vi "SprachEditor.vi"() -> ()   [LabVIEW 2020, in "Sprachverwaltung.lvlib"]
uses:
  Sprachverwaltung.lvlib
  Allgemein/Sprachauswahl native.ctl
  Visualisierungs Elemente/Button.ctl
  Seiten.ctl
  FGV Aktion Tabelle zerlegen.ctl
  Seiten/System Einstellungen V2/Aktioen FGV System Konstanten.ctl
  Allgemein/allgemeine Sub-VIs.lvlib
  Seiten/System Einstellungen V2/System Einstellungen V2.lvlib
panel:
  in  "Registerkarte":enum32{"Deutsch", "English"}(tab)
  out "Deutsch":string[](array[string])
  out "English":string[](array[string]) caption="Englisch"
  in  "Bearbeitungsspalte":string[](array[string])
  in  "Seiten":T1 caption="Seiten:"
  in  "Save":T2 caption="Abbrechen"
  in  "Cancel":T2 caption="Abbrechen"
  in  "Sprache":T3 caption="Bitte wählen Sie eine Sprache:" items=["Français"=2, "Italiano"=3, "Castellano"=4, "Polski"=5]
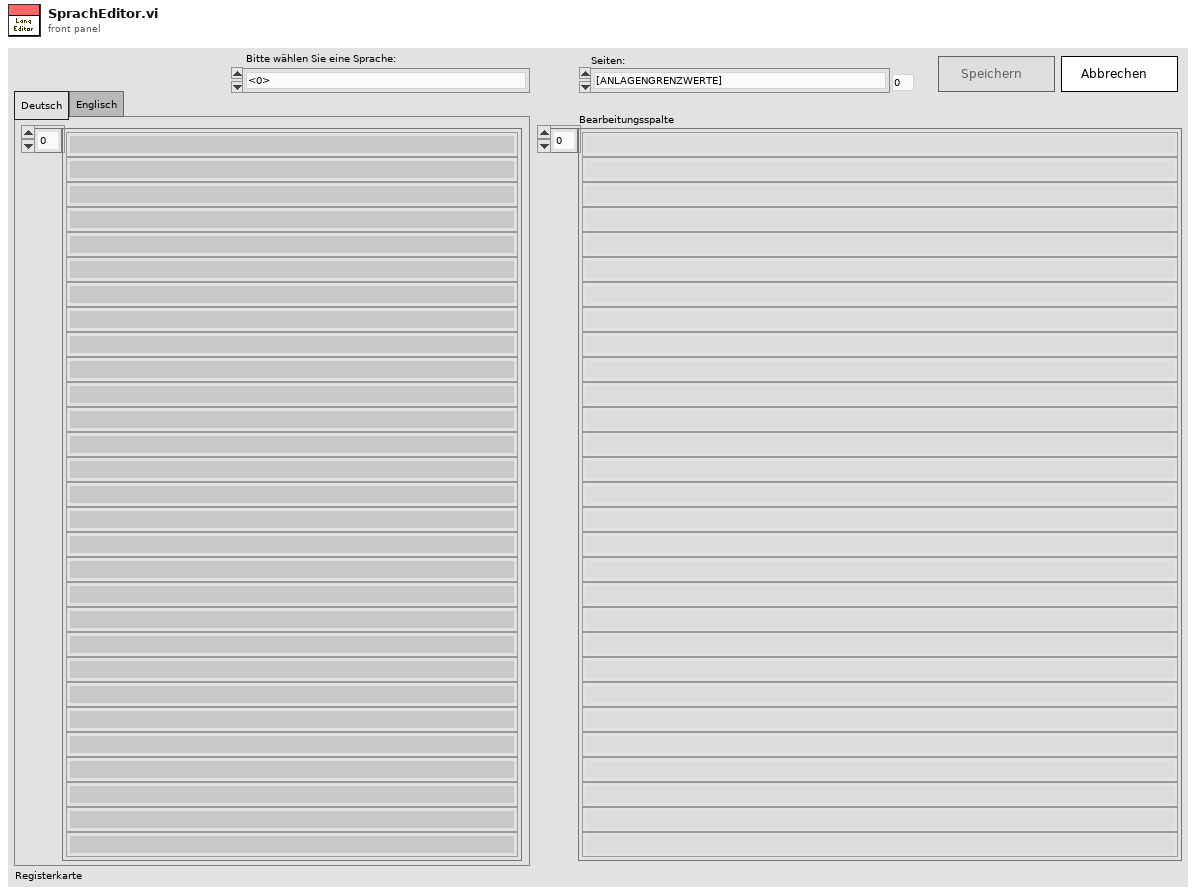
[diagram p1: front panel]
types:
  T1 = typedef "Sprachverwaltung.lvlib/Seiten.ctl" = enum16{"[ANLAGENGRENZWERTE]", "[LOG KONFIG]", "[GASZUORDNUNG]", "[ANLAGENÜBERSICHT]", "[GRAFIK]", "[CONFIG DIAGRAMME]", "[KONFIGURATION FTIR]", "[GASLISTE VERGLEICHEN]", "[ALGEBRAIC KONFIG]", "[FTIR DIAGNOSE]", "[ERWEITERTE KONFIG]", "[KONFIG AK]", "[STATUS STEUERUNG]", "[PID PARAMETER DRUCK-REGLER]", "[DICHTHEITSTEST]", "[T90 KONFIG]", "[T90]", "[HINTERGRUND]", "[SYSTEM EINSTELLUNGEN V2]", "[COPYRIGHT]", "[STATUSÜBERSICHT]", "[PASSWORTVERWALTUNG]", "[PASSWORT AENDERN]", "[FUNKTIONSTASTEN]", "[PNS]", "[DIAG PNS]", "[RUNTIME MENUE]", "[FAS06]", "[PERMANENT BEREICH]", "[RUNTIME BEENDEN]", "[SPEICHERN]", "[STOERMELDUNGEN]", "[STOERMELDEPUFFER]", "[STOERMELDE-KONFIG]", "[STOERMELDUNGSDATEI]", "[ERWEITERTE GASLISTE]", "[LINEARISIERUNG FTIR]", "[ARN TEST]", "[ARN PROTOKOLL]", "[FEHLER STEUERUNG]", "[POLYNOMKOEFFIZIENTEN]", "[KONFIG LINEARITY VERIFICATION]", "[AUTO LIN VERIFICATION]", "[GRAPHIK KURVEN]", "[EPA DICHTHEITSTEST]", "[REZEPT LADEN]", "[REZEPTWECHSEL]", "[DIAG ZYKLUSZEIT]", "[EPA KONTROLLE PARAMETER]", "[KONFIG GASTEILER]", "[KALIBRIERDATEN LADEN]", "[KONTROLLE PARAMETER VOR LIN]", "[KONFIGURATION KALIBRIERGASE]", "[INTERFERENCE VERIFICATION]", "[INTERFERENCE VERIFICATION 375]", "[INTERFERENCE PROTOKOLL 375]", "[INTERFERENCE PROTOKOLL]", "[INTERFERENCE HILFE]", "[SPUELEN]", "[GASTEILER SPUELEN]", "[GASTEILER KALIBRIEREN]", "[SENSOR KONFIGURATION]", "[KONFIGURATION PMA]", "[KALIBRIERDATEN]", "[KONFIGURATION FID]", "[ABB MANUELL KALIBRIEREN]", "[PMA MANUELL KALIBRIEREN]", "[SPRACHAUSWAHL]", "[SYS LOG HISTORY]", "[SYS LOG STATUS]", "[PNS UEBERSICHT]\t", "[CG TEST]", "[KONFIG CG CHECK]", "[HOVA MAIN]", "[HORIBA GDC]", "[BACKUP]", "[SPAN FAKTOREN]", "[CG POPUP]", "[AUTO CALIBRATION]", "[LIN V2]", "[O2 LEAKTEST]", "[CG TEST RESULT]", "[GASTEILER ABWEICHUNG]", "[EPA LIN CHECK PROTOKOLL]", "[LIN CHECK PROTOKOLL]", "[LEAK CHECK PROTOKOLL]", "[O2 LEAK PROTOKOLL]", "[HANG UP PROTOKOLL]", "[T90 PROTOKOLL]", "[SPRACHEDITOR]", "[SYSLOG CRIO MESSAGES]", "[SYSLOG PC MESSAGES]", "[SYSLOG PROPERTIES MESSAGES]", "[T90 EPA]", "[T90 EPA PDF]", "[SCHEDULER]", "[HINTERGRUND V2]", "[CG TEST PDF]", "[CHILLER EPA TEST]", "[CHILLER EPA PROTOKOLL]", "[FID O2 EPA TEST]", "[FID O2 EPA PROTOKOLL]", "[DRIFT EPA TEST]", "[DRIFT EPA PROTOKOLL]", "[PRE EPA TEST]", "[PRE EPA PROTOKOLL]", "[FID OPTIMIZATION]", "[FID OPTIMIZATION PDF]", "[FID RESPONSE FAKTOR]"}
  T2 = typedef "Button.ctl" = bool
  T3 = typedef "Sprachverwaltung.lvlib/Sprachauswahl native.ctl" = u16
  T4 = typedef "Sprachverwaltung.lvlib/FGV Aktion Tabelle zerlegen.ctl" = enum16{"laden", "vereinzeln", "speichern"}
  T5 = enum8{"Enabled", "Disabled", "Disabled and Grayed Out"}
  T6 = typedef "LVStringsAndValuesArrayTypeDef_U16.ctl" = cluster{"String":string, "Value":u16}[]
  T7 = typedef "System Einstellungen V2.lvlib/Aktioen FGV System Konstanten.ctl" = enum16{"lesen", "laden", "speichern", "Sprache"}
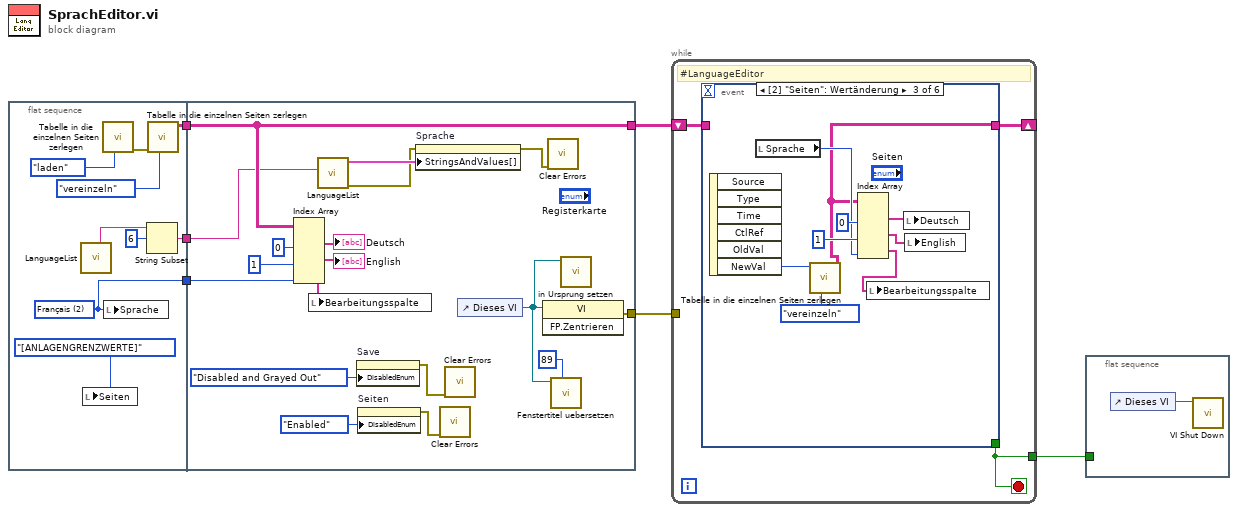
[diagram p0: block diagram]
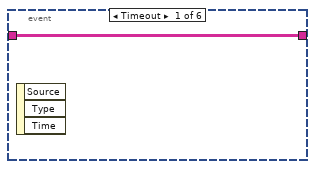
[diagram p2: hidden frame]
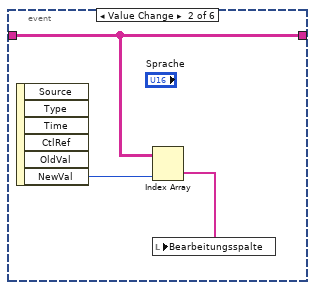
[diagram p3: hidden frame]
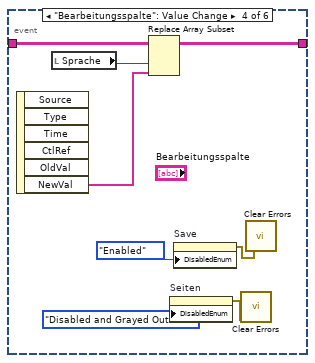
[diagram p4: hidden frame]
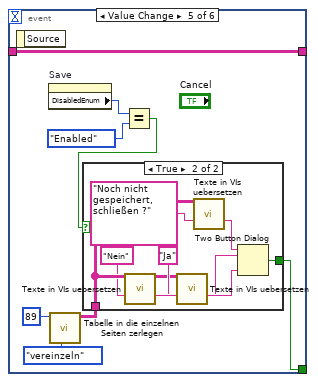
[diagram p5: hidden frame]
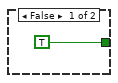
[diagram p6: hidden frame]
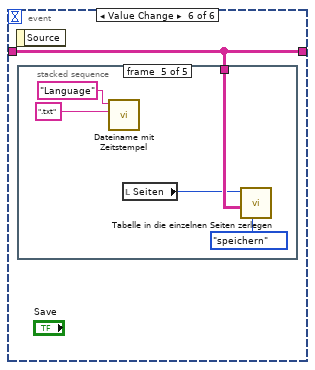
[diagram p7: hidden frame]
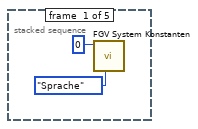
[diagram p8: hidden frame]
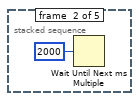
[diagram p9: hidden frame]
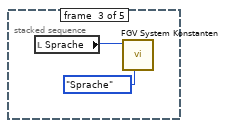
[diagram p10: hidden frame]
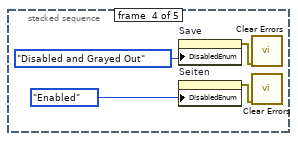
[diagram p11: hidden frame]
diagram:
  n1 = flat-sequence {
    tunnel: [w12] -> w3
    tunnel: [w9] -> w2
    tunnel: [w7] -> w1
    tunnel: [w30] -> w6
    tunnel: [w29] -> w4
    tunnel: w3 -> [w29]
    tunnel: w2 -> [w28]
    tunnel: w1 -> [w23]
    frame #0 {
      w7 = T3 2 items=["Deutsch", "English", "Français", "Italiano", "Castellano", "Polski"] ("Sprache")
      n2 = call "LanguageList.vi"() -> ("FullLanguageList"=w11:string)  [unwired: 6 in, 5 out]
      n3 = local write "Seiten"(Seiten."[ANLAGENGRENZWERTE]" ("Seiten")) -> ()
      n4 = call "Tabelle in die einzelnen Seiten zerlegen.vi"("Aktion"=FGV_Aktion_Tabelle_zerlegen."laden") -> ("error out"=w13:errorcluster)  [unwired: 8 in, 2 out]
      n5 = local write "Sprache"(w7) -> ()
      n6 = String Subset(string=w11, offset (0)=6 ("Offset (0)")) -> (substring=w9:string)  [unwired: 1 in]
      n7 = call "Tabelle in die einzelnen Seiten zerlegen.vi"("Aktion"=FGV_Aktion_Tabelle_zerlegen."vereinzeln", "error in (no error)"=w13) -> ("Sprachliste"=w12:string[][])  [unwired: 7 in, 2 out]
    }
    frame #1 {
      n8 = Index Array(array=w29, index (col) #1=0 ("Deaktivierter Index (Spalte)"), index (col) #2=1 ("Index (Spalte)"), index (col) #3=w23) -> (element #1=→"Deutsch":string[], element #2=→"English":string[], element #3=w22:string[])  [unwired: 3 in]
      n9 = local write "Bearbeitungsspalte"(w22) -> ()
      n10 = call "LanguageList.vi"("LanguageList"=w28) -> ("Fehler (Ausgang)"=w32:errorcluster, "Strings und Werte []"=w33:T6)  [unwired: 5 in, 4 out]
      n11 = property on="Save" class="Bool."("DisabledEnum"=T5."Disabled and Grayed Out" ("Deaktiviert")) -> (error out=w20:errorcluster)  [unwired: 2 in, 1 out]
      n12 = property on="Seiten" class="Enum (strikt)"("DisabledEnum"=T5."Enabled" ("Deaktiviert")) -> (error out=w18:errorcluster)  [unwired: 2 in, 1 out]
      n13 = property on="Sprache" class="Ring (strikt)"(error in=w32, "StringsAndValues[]"=w33) -> (error out=w31:errorcluster)  [unwired: 1 in, 1 out]
      n14 = call <vilib>:"Clear Errors.vi"("error in (no error)"=w18) -> ()  [unwired: 5 in, 2 out]
      n15 = call <vilib>:"Clear Errors.vi"("error in (no error)"=w20) -> ()  [unwired: 5 in, 2 out]
      n16 = control-ref of="Dieses VI"() -> (w16:refnum<vi>)
      n17 = invoke class="VI" method="FP.Zentrieren"(reference=w16) -> (error out=w30:errorcluster)  [unwired: 2 in, 2 out]
      n18 = call <vilib>:"Clear Errors.vi"("error in (no error)"=w31) -> ()  [unwired: 5 in, 2 out]
      n19 = call "Fenstertitel uebersetzen.vi"("Index (Seite)"=89, "Dieses VI"=w16) -> ()  [unwired: 6 in, 4 out]
      n20 = call "in Ursprung setzen.vi"("VI Referenz"=w16) -> ()  [unwired: 10 in, 1 out]
    }
  }
  n21 = while {
    tunnel: w6 -> [_]
    tunnel: [w36] -> w5
    shift-right: [w34] -> _
    shift-left: w4 -> [w35]
    stop <- w36 stop-if-true
    # "#LanguageEditor"
    n22 = event shown="[2] \"Seiten\": Wertänderung" {
      selector: _ -> [_ _ _ _ _ _]
      dyn-events: _ -> [_ _ _ _ _ _]
      timeout: _ -> [_ _ _ _ _ _]
      tunnel: [_ _ _ _ w65 _] -> w36
      tunnel: w35 -> [w37 w40 _ w53 w64 w76]
      tunnel: [w37 w40 w41 w52 w64 w76] -> w34
      event Timeout {
        n23 = event-data() -> ()  [unwired: 1 in, 3 out]
      }
      event Value Change {
        n24 = event-data() -> ("NewVal"=w38:T3)  [unwired: 1 in, 5 out]
        n25 = Index Array(array=w40, index (col)=w38) -> (element=w39:string[])  [unwired: 1 in]
        n26 = local write "Bearbeitungsspalte"(w39) -> ()
      }
      event Value Change {
        n27 = event-data() -> ("NewVal"=w48:T1)  [unwired: 1 in, 5 out]
        n28 = local read "Sprache"() -> (w42:T3)
        n29 = call "Tabelle in die einzelnen Seiten zerlegen.vi"("Aktion"=FGV_Aktion_Tabelle_zerlegen."vereinzeln", "Index (Seite)"=w48) -> ("Sprachliste"=w41:string[][])  [unwired: 7 in, 2 out]
        n30 = Index Array(array=w41, index (col) #1=0 ("Deaktivierter Index (Spalte)"), index (col) #2=1 ("Index (Spalte)"), index (col) #3=w42) -> (element #1=w45:string[], element #2=w44:string[], element #3=w43:string[])  [unwired: 3 in]
        n31 = local write "Bearbeitungsspalte"(w43) -> ()
        n32 = local write "Deutsch"(w45) -> ()
        n33 = local write "English"(w44) -> ()
      }
      event "Bearbeitungsspalte": Value Change {
        n34 = event-data() -> ("NewVal"=w50:string[])  [unwired: 1 in, 5 out]
        n35 = local read "Sprache"() -> (w51:T3)
        n36 = Replace Array Subset(array=w53, new element=w50, index (col)=w51) -> (w52:string[][])  [unwired: 1 in]
        n37 = property on="Seiten" class="Enum (strikt)"("DisabledEnum"=T5."Disabled and Grayed Out" ("Deaktiviert")) -> (error out=w54:errorcluster)  [unwired: 2 in, 1 out]
        n38 = property on="Save" class="Bool."("DisabledEnum"=T5."Enabled" ("Deaktiviert")) -> (error out=w57:errorcluster)  [unwired: 2 in, 1 out]
        n39 = call <vilib>:"Clear Errors.vi"("error in (no error)"=w54) -> ()  [unwired: 5 in, 2 out]
        n40 = call <vilib>:"Clear Errors.vi"("error in (no error)"=w57) -> ()  [unwired: 5 in, 2 out]
      }
      event Value Change {
        n41 = event-data() -> ()  [unwired: 1 in, 1 out]
        n42 = property on="Save" class="Bool."() -> ("DisabledEnum"=w63:T5)  [unwired: 2 in, 2 out]
        n43 = call "Tabelle in die einzelnen Seiten zerlegen.vi"("Aktion"=FGV_Aktion_Tabelle_zerlegen."vereinzeln", "Index (Seite)"=89) -> ("Sprachliste"=w58:string[][])  [unwired: 7 in, 2 out]
        n44 = Equal?(x=w63, y=T5."Enabled" ("Deaktiviert")) -> (x = y?=w61:bool)
        n45 = case shown="True" w61 {
          tunnel: [TRUE ("T button?") w75] -> w65
          tunnel: w58 -> [_ w72]
          frame False {
          }
          frame True {
            n46 = call "Texte in VIs uebersetzen.vi"("Sprachliste"=w72, "String zum Übersetzen"="Nein" ("Text für F-Schaltfläche (\"Abbrechen\")")) -> ("Sprachliste out"=w67:string[][], "String zum Übersetzen"=w70:string)  [unwired: 9 in, 3 out]
            n47 = call "Texte in VIs uebersetzen.vi"("Sprachliste"=w67, "String zum Übersetzen"="Ja" ("Text für T-Schaltfläche (\"OK\")")) -> ("String zum Übersetzen"=w68:string)  [unwired: 9 in, 4 out]
            n48 = call "Texte in VIs uebersetzen.vi"("Sprachliste"=w72, "String zum Übersetzen"="Noch nicht  gespeichert, schließen ?" ("Nachricht")) -> ("String zum Übersetzen"=w73:string)  [unwired: 9 in, 4 out]
            n49 = Two Button Dialog(message=w73, 1:w70, 2:w68) -> (T button?=w75:bool)
          }
        }
      }
      event Value Change {
        n50 = event-data() -> ()  [unwired: 1 in, 1 out]
        n51 = stacked-sequence {
          tunnel: w76 -> [_ _ _ _ w90]
          frame #0 {
            n52 = call "FGV System Konstanten.vi"("Aktionen"=Aktioen_FGV_System_Konstanten."Sprache", "Sprache"=u32 0) -> ()  [unwired: 5 in, 5 out]
          }
          frame #1 {
            n53 = Wait Until Next ms Multiple(millisecond multiple=u32 2000 ("ms")) -> ()  [unwired: 1 out]
          }
          frame #2 {
            n54 = local read "Sprache"() -> (w80:T3)
            n55 = call "FGV System Konstanten.vi"("Aktionen"=Aktioen_FGV_System_Konstanten."Sprache", "Sprache"=w80) -> ()  [unwired: 5 in, 5 out]
          }
          frame #3 {
            n56 = property on="Save" class="Bool."("DisabledEnum"=T5."Disabled and Grayed Out" ("Deaktiviert")) -> (error out=w83:errorcluster)  [unwired: 2 in, 1 out]
            n57 = property on="Seiten" class="Enum (strikt)"("DisabledEnum"=T5."Enabled" ("Deaktiviert")) -> (error out=w85:errorcluster)  [unwired: 2 in, 1 out]
            n58 = call <vilib>:"Clear Errors.vi"("error in (no error)"=w83) -> ()  [unwired: 5 in, 2 out]
            n59 = call <vilib>:"Clear Errors.vi"("error in (no error)"=w85) -> ()  [unwired: 5 in, 2 out]
          }
          frame #4 {
            n60 = call "Dateiname mit Zeitstempel.vi"("Extension in"=".txt" ("alternative Datei"), "File Name in"="Language" ("alternative Datei")) -> ()  [unwired: 9 in, 1 out]
            n61 = local read "Seiten"() -> (w88:T1)
            n62 = call "Tabelle in die einzelnen Seiten zerlegen.vi"("Aktion"=FGV_Aktion_Tabelle_zerlegen."speichern", "Sprachseite"=w90, "Index (Seite)"=w88) -> ()  [unwired: 6 in, 3 out]
          }
        }
      }
    }
  }
  n63 = flat-sequence {
    tunnel: w5 -> [_]
    frame #0 {
      n64 = control-ref of="Dieses VI"() -> (w91:refnum<vi>)
      n65 = call "VI Shut Down.vi"("VI Referenz"=w91) -> ()  [unwired: 11 in]
    }
  }
